vi "writeI16.vi"(8 "error in (no error)":errorcluster, 10 "Input":i16, 11 "M1M3SAL in":refnum<class "M1M3SAL.lvclass">) -> (0 "error out":errorcluster, 3 "M1M3SAL out":refnum<class "M1M3SAL.lvclass">)   [LabVIEW 2016, in "M1M3SupportCommunicator.lvlib" / "M1M3SAL.lvclass"]
uses:
  M1M3SAL.lvclass
  M1M3SAL.lvclass/M1M3SAL.ctl
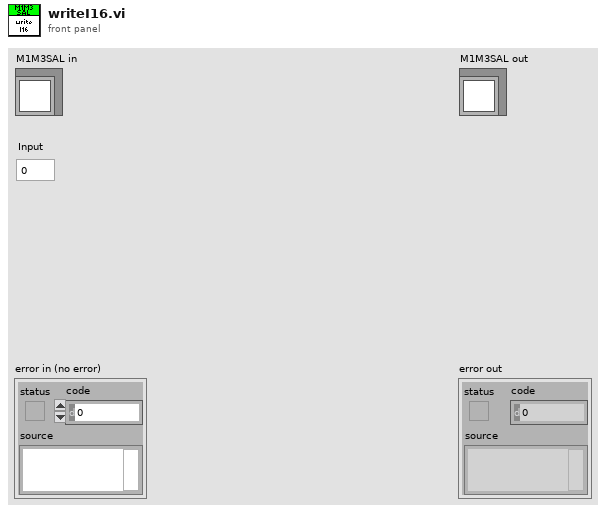
[diagram p1: front panel]
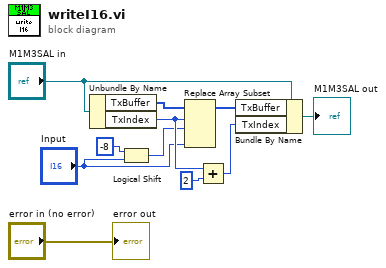
[diagram p0: block diagram]
diagram:
  n1 = Unbundle By Name("M1M3SAL in") -> ("TxBuffer"=w9:u8[], "TxIndex"=w8:i32)
  n2 = Logical Shift(y=i16 -8, x="Input") -> (x << y=w2:i16)
  n3 = Replace Array Subset(array=w9, new element #1=w2, index #1=w8, new element #2="Input") -> (w5:u8[])  [unwired: 1 in]
  n4 = Add(x=w8, y=2) -> (x+y=w6:i32)
  n5 = Bundle By Name(cluster="M1M3SAL in", "TxBuffer"=w5, "TxIndex"=w6) -> (→"M1M3SAL out":refnum<class "M1M3SAL.lvclass">)
  "error out" <- "error in (no error)"
